vi "5BLABVIEW (1).vi"() -> ()   [LabVIEW 2013]
panel:
  in  "stop":bool
  out "Lissajious figurs":cluster{"Y":dbl[], "Y":dbl[]}[](graph)
  in  "Phase 2":dbl(knob) scale=0.0..360.0
  in  "Frequency 2":dbl(knob) scale=0.0..50.0
  in  "Amplitude 2":dbl(knob) scale=0.0..50.0
  in  "Phase":dbl(knob) scale=0.0..360.0
  in  "Frequency":dbl(knob) scale=0.0..50.0
  in  "Amplitude":dbl(knob) scale=0.0..50.0
  # "5(b).GENERATION OF LISSAJOUS FIGURES USING LABVIEW"
  # "O.SRINIVAS\n23A91A04H6"
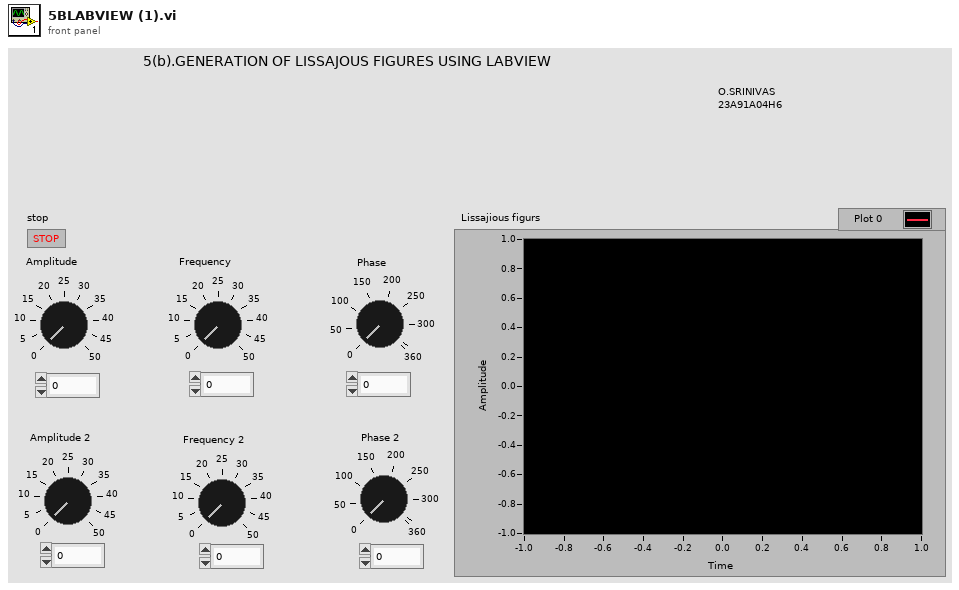
[diagram p1: front panel]
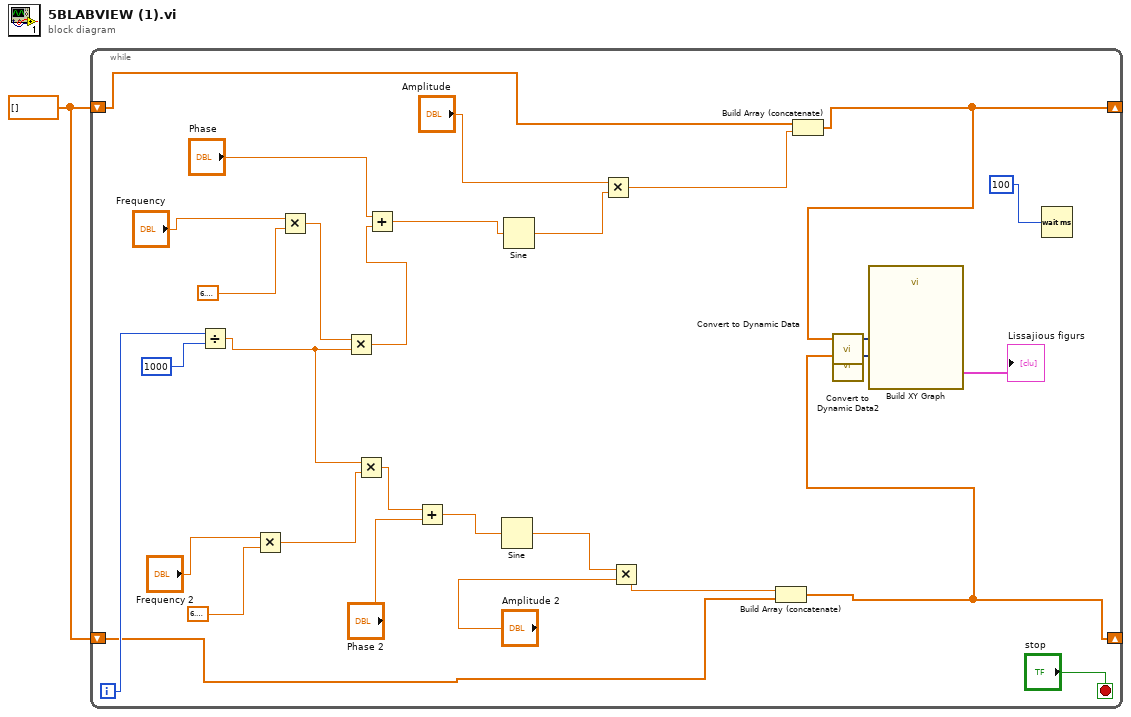
[diagram p0: block diagram]
diagram:
  w1 = dbl[] []
  n1 = while {
    shift-right: [w7] -> _
    shift-left: w1 -> [w9]
    shift-right: [w5] -> _
    shift-left: w1 -> [w11]
    i -> [w26]
    stop <- "stop" stop-if-true
    n2 = Divide(x=w26, y=1000) -> (x/y=w22:dbl)
    n3 = Multiply(x="Frequency 2", y=6.283185307179586 ("Pi Multiplied By 2")) -> (x*y=w23:dbl)
    n4 = Multiply(x="Frequency", y=6.283185307179586 ("Pi Multiplied By 2")) -> (x*y=w24:dbl)
    n5 = Multiply(x=w24, y=w22) -> (x*y=w21:dbl)
    n6 = Multiply(x=w22, y=w23) -> (x*y=w18:dbl)
    n7 = Add(x="Phase", y=w21) -> (x+y=w15:dbl)
    n8 = Add(x=w18, y="Phase 2") -> (x+y=w13:dbl)
    n9 = Sine(x=w13) -> (sin(x)=w12:dbl)
    n10 = Sine(x=w15) -> (sin(x)=w14:dbl)
    n11 = Multiply(x="Amplitude", y=w14) -> (x*y=w8:dbl)
    n12 = Multiply(x=w12, y="Amplitude 2") -> (x*y=w10:dbl)
    n13 = Build Array (concatenate) "Build Array"(w10, w11) -> (w5:dbl[])
    n14 = Build Array (concatenate)(w9, w8) -> (w7:dbl[])
    n15 = call "Convert to Dynamic Data"("Array"=w7) -> ("Dynamic Data Type"=w6:dynamicdata)  [unwired: 3 in]
    n16 = call "Convert to Dynamic Data2"("Array"=w5) -> ("Dynamic Data Type"=w4:dynamicdata)  [unwired: 3 in]
    n17 = call "Build XY Graph"("Y Input"=w4, "X Input"=w6) -> ("XY Graph"=→"Lissajious figurs":cluster{"X":dbl[], "Y":dbl[]}[])  [unwired: 8 in, 1 out]
    n18 = Wait (ms)(milliseconds to wait=u32 100) -> ()  [unwired: 1 out]
  }
